vi "LakeShore 370 Zones.vi"() -> ()   [LabVIEW 2021]
doc: "This VI manages the zones for the LakeShore Model 370 Temperature Controller. Set the address and run the VI. The current values are read and entered into the table. Add any additional values or edit the current values, you do not need to sort by temperature. When the OK button is pressed the values are sorted and uploaded. The indicators will tell you which zones have been updated.\n\nScott Hannahs, <sth@magnet.fsu.edu> NHMFL-FSU, May 2003"
panel:
  out "Updated":bool[](array[boolean])
  in  "OK Button":bool
  in  "VISA session":refnum<visa-resource-name>
  in  "Zone List":T1(array[cluster]) {"Analog 2 Output (0.000)" min=-100.0 max=100.0 step=0.001 format="%.1f"; "Analog 1 Output (0.000)" min=-100.0 max=100.0 step=0.001 format="%.1f"; "Relay High (0: Off)" items=["Off", "On"]; "Relay Low (0: Off)" items=["Off", "On"]; "Heater Range (0: Off)" items=["Off", "31.6 uA", "100 uA", "316 uA", "1.00 mA", "3.16 mA", "10.0 mA", "31.6 mA", "100 mA"]; "Manual" format="%.1f"; "D" format="%.1f"; "I" format="%.1f"; "P" format="%.3f"; "Limit" format="%.3f"}
  # "The Limit starts at 0K and the limit is the upper limit for the zone.  The data can be entered in any order and will be sorted by the Limit value before it is sent to the LakeShore 370."
  # "Relay\nLow  High"
  # "Zone #"
  # "Limit (K)"
  # "P"
  # "I (sec)"
  # "D (sec)"
  # "Manual"
  # "Range"
  # "Analog 1(%)"
  # "Analog 2(%)"
  # "1"
  # "2"
  # "3"
  # "4"
  # "5"
  # "6"
  # "7"
  # "8"
  # "9"
  # "10"
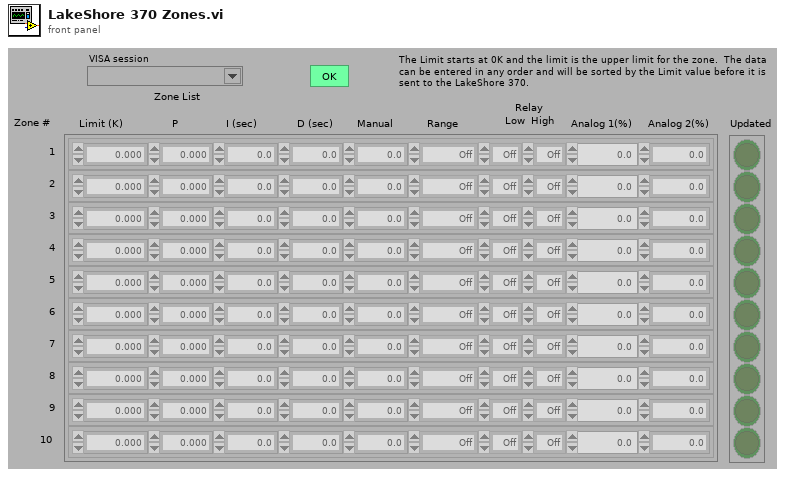
[diagram p1: front panel]
types:
  T1 = cluster{"Limit":dbl, "P":dbl, "I":dbl, "D":dbl, "Manual":dbl, "Heater Range (0: Off)":dbl, "Relay Low (0: Off)":dbl, "Relay High (0: Off)":dbl, "Analog 1 Output (0.000)":dbl, "Analog 2 Output (0.000)":dbl}[]
  T2 = cluster{"Measurement[0]":dbl, "Measurement[1]":dbl, "Measurement[2]":dbl, "Measurement[3]":dbl, "Measurement[4]":dbl, "Measurement[5]":dbl, "Measurement[6]":dbl, "Measurement[7]":dbl, "Measurement[8]":dbl, "Measurement[9]":dbl}
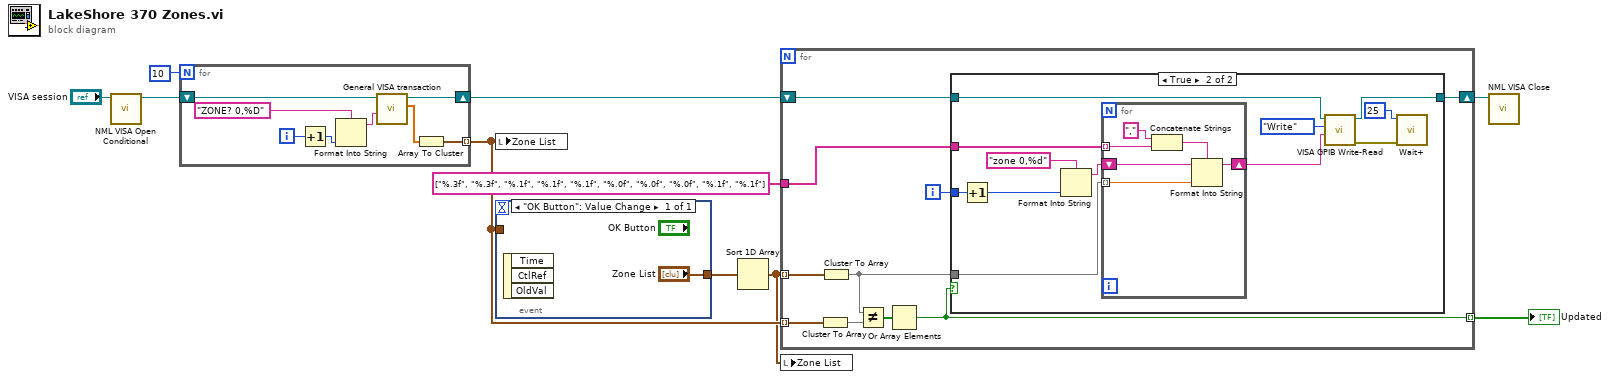
[diagram p0: block diagram]
diagram:
  n1 = call "NML VISA Open Conditional.vi"("VISA resource name"="VISA session") -> ("dup VISA Session"=w2:refnum<visa-resource-name>)  [unwired: 8 in, 2 out]
  n2 = for {
    N: 10 -> [_]
    tunnel: [w12] -> w6 mode=indexing
    shift-right: [w11] -> w3
    shift-left: w2 -> [w14]
    i -> [w18]
    n3 = Increment(x=w18) -> (x+1=w16:i32)
    n4 = Format Into String(format string="ZONE? 0,%D", w16) -> (resulting string=w15:string)  [unwired: 2 in, 1 out]
    n5 = call "General VISA transaction.vi"("Command String"=w15, "VISA Session"=w14) -> ("Measurement"=w13:dbl[], "dup VISA Session"=w11:refnum<visa-resource-name>)  [unwired: 4 in, 4 out]
    n6 = Array To Cluster(array=w13) -> (cluster=w12:T2)
  }
  n7 = local write "Zone List"(w6) -> ()
  n8 = event shown="[0] \"OK Button\": Value Change" {
    selector: _ -> [_]
    dyn-events: _ -> [_]
    timeout: _ -> [_]
    tunnel: ["Zone List"] -> w8
    tunnel: w6 -> [_]
    event "OK Button": Value Change {
      n9 = event-data() -> ()  [unwired: 1 in, 3 out]
    }
  }
  n10 = Sort 1D Array(array=w8) -> (sorted array=w4:T1)
  n11 = for {
    tunnel: w4 -> [w29] mode=indexing
    tunnel: string[] ["%.3f", "%.3f", "%.1f", "%.1f", "%.1f", "%.0f", "%.0f", "%.0f", "%.1f", "%.1f"] -> [w26]
    tunnel: w6 -> [w25] mode=indexing
    tunnel: [w22] -> w5 mode=indexing
    shift-right: [w20] -> w1
    shift-left: w3 -> [w21]
    i -> [w27]
    n12 = Cluster To Array(cluster=w25) -> (array=w24:dbl[])
    n13 = Cluster To Array(cluster=w29) -> (array=w28:dbl[])
    n14 = Not Equal?(x=w28, y=w24) -> (x != y?=w23:bool[])
    n15 = Or Array Elements(Boolean array=w23) -> (logical OR=w22:bool)
    n16 = case shown="True" w22 {
      tunnel: w28 -> [_ w42]
      tunnel: w27 -> [_ w41]
      tunnel: w26 -> [_ w37]
      tunnel: w21 -> [w30 w32]
      tunnel: [w30 w31] -> w20
      frame False {
      }
      frame True {
        n17 = Increment(x=w41) -> (x+1=w40:i32)
        n18 = Format Into String(format string="zone 0,%d", w40) -> (resulting string=w38:string)  [unwired: 2 in, 1 out]
        n19 = for {
          tunnel: w42 -> [w47] mode=indexing
          shift-right: [w46] -> w36
          shift-left: w38 -> [w48]
          tunnel: w37 -> [w44] mode=indexing
          n20 = Concatenate Strings("," ("string"), w44) -> (w45:string)
          n21 = Format Into String(format string=w45, initial string=w48, w47) -> (resulting string=w46:string)  [unwired: 1 in, 1 out]
        }
        n22 = call "VISA GPIB Write-Read.vi"("Command"=w36, "Action"=enum16{"Write", "Read", "Write & Read"}."Write", "VISA resource name"=w32) -> ("error out"=w34:errorcluster, "dup VISA Session"=w31:refnum<visa-resource-name>)  [unwired: 5 in, 2 out]
        n23 = call "Wait+.vi"("Error In"=w34, "milliseconds to wait"=u32 25) -> ()  [unwired: 4 in, 2 out]
      }
    }
  }
  "Updated" <- w5
  n24 = local write "Zone List"(w4) -> ()
  n25 = call "NML VISA Close.vi"("VISA resource name"=w1) -> ()  [unwired: 10 in, 1 out]
